vi "Industri Kerupuk Kentang.vi"() -> ()   [LabVIEW 2021]
uses:
  Control 12.ctl
panel:
  out "Proses Packing Selesai":bool
  out "Pencampuran Kentang \ndengan bumbu":bool
  out "Kompor Menyala":bool
  out "Keran 2 Menyala":bool
  out "Proses Pemotongan Kentang":bool
  out "Conveyor 2":dbl(slide)=10.0 scale=0.0..10.0
  out "Closer":dbl(slide) scale=0.0..10.0
  out "Conveyor":dbl(slide)=10.0 scale=0.0..10.0
  out "Pengadukan Bumbu":bool
  out "Pengeringan Bumbu":bool
  out "Tangki Bumbu":dbl(slide) scale=0.0..150.0
  out "Suhu Oven":dbl(slide) scale=0.0..150.0
  out "Silinder single acting":dbl(slide) scale=0.0..2.0
  out "Proximity":bool
  out "Silinder Pemotong 2":dbl(slide) scale=0.0..1.0
  out "Conveyor  2":dbl(slide) scale=0.0..1000.0
  out "Valve":T1
  out "Tachometer":dbl(knob) scale=0.0..250.0
  out "Tangki Minyak":dbl(slide) scale=0.0..1000.0
  out "Tangki Air":dbl(slide) scale=0.0..1000.0
  out "Tangki Penggorengan":dbl(slide) scale=0.0..180.0
  out "Pengukuran berat Kentang":bool
  out "Conveyor  1":dbl(slide) scale=0.0..35.0
  out "Tangki Pencucian":dbl(slide) scale=0.0..180.0
  out "Keran 1 menyala":bool
  out "Suhu Kompor Penggorengan":dbl(slide) scale=0.0..120.0
  out "Kecepatan pengaduk":dbl(knob) scale=0.0..100.0
  out "Berat Kentang":dbl(knob) scale=0.0..100.0
  # "1. Mesin Pengupas Kentang\n(Potato Peeler)"
  # "rpm"
  # "Packing Kerupuk Kentang"
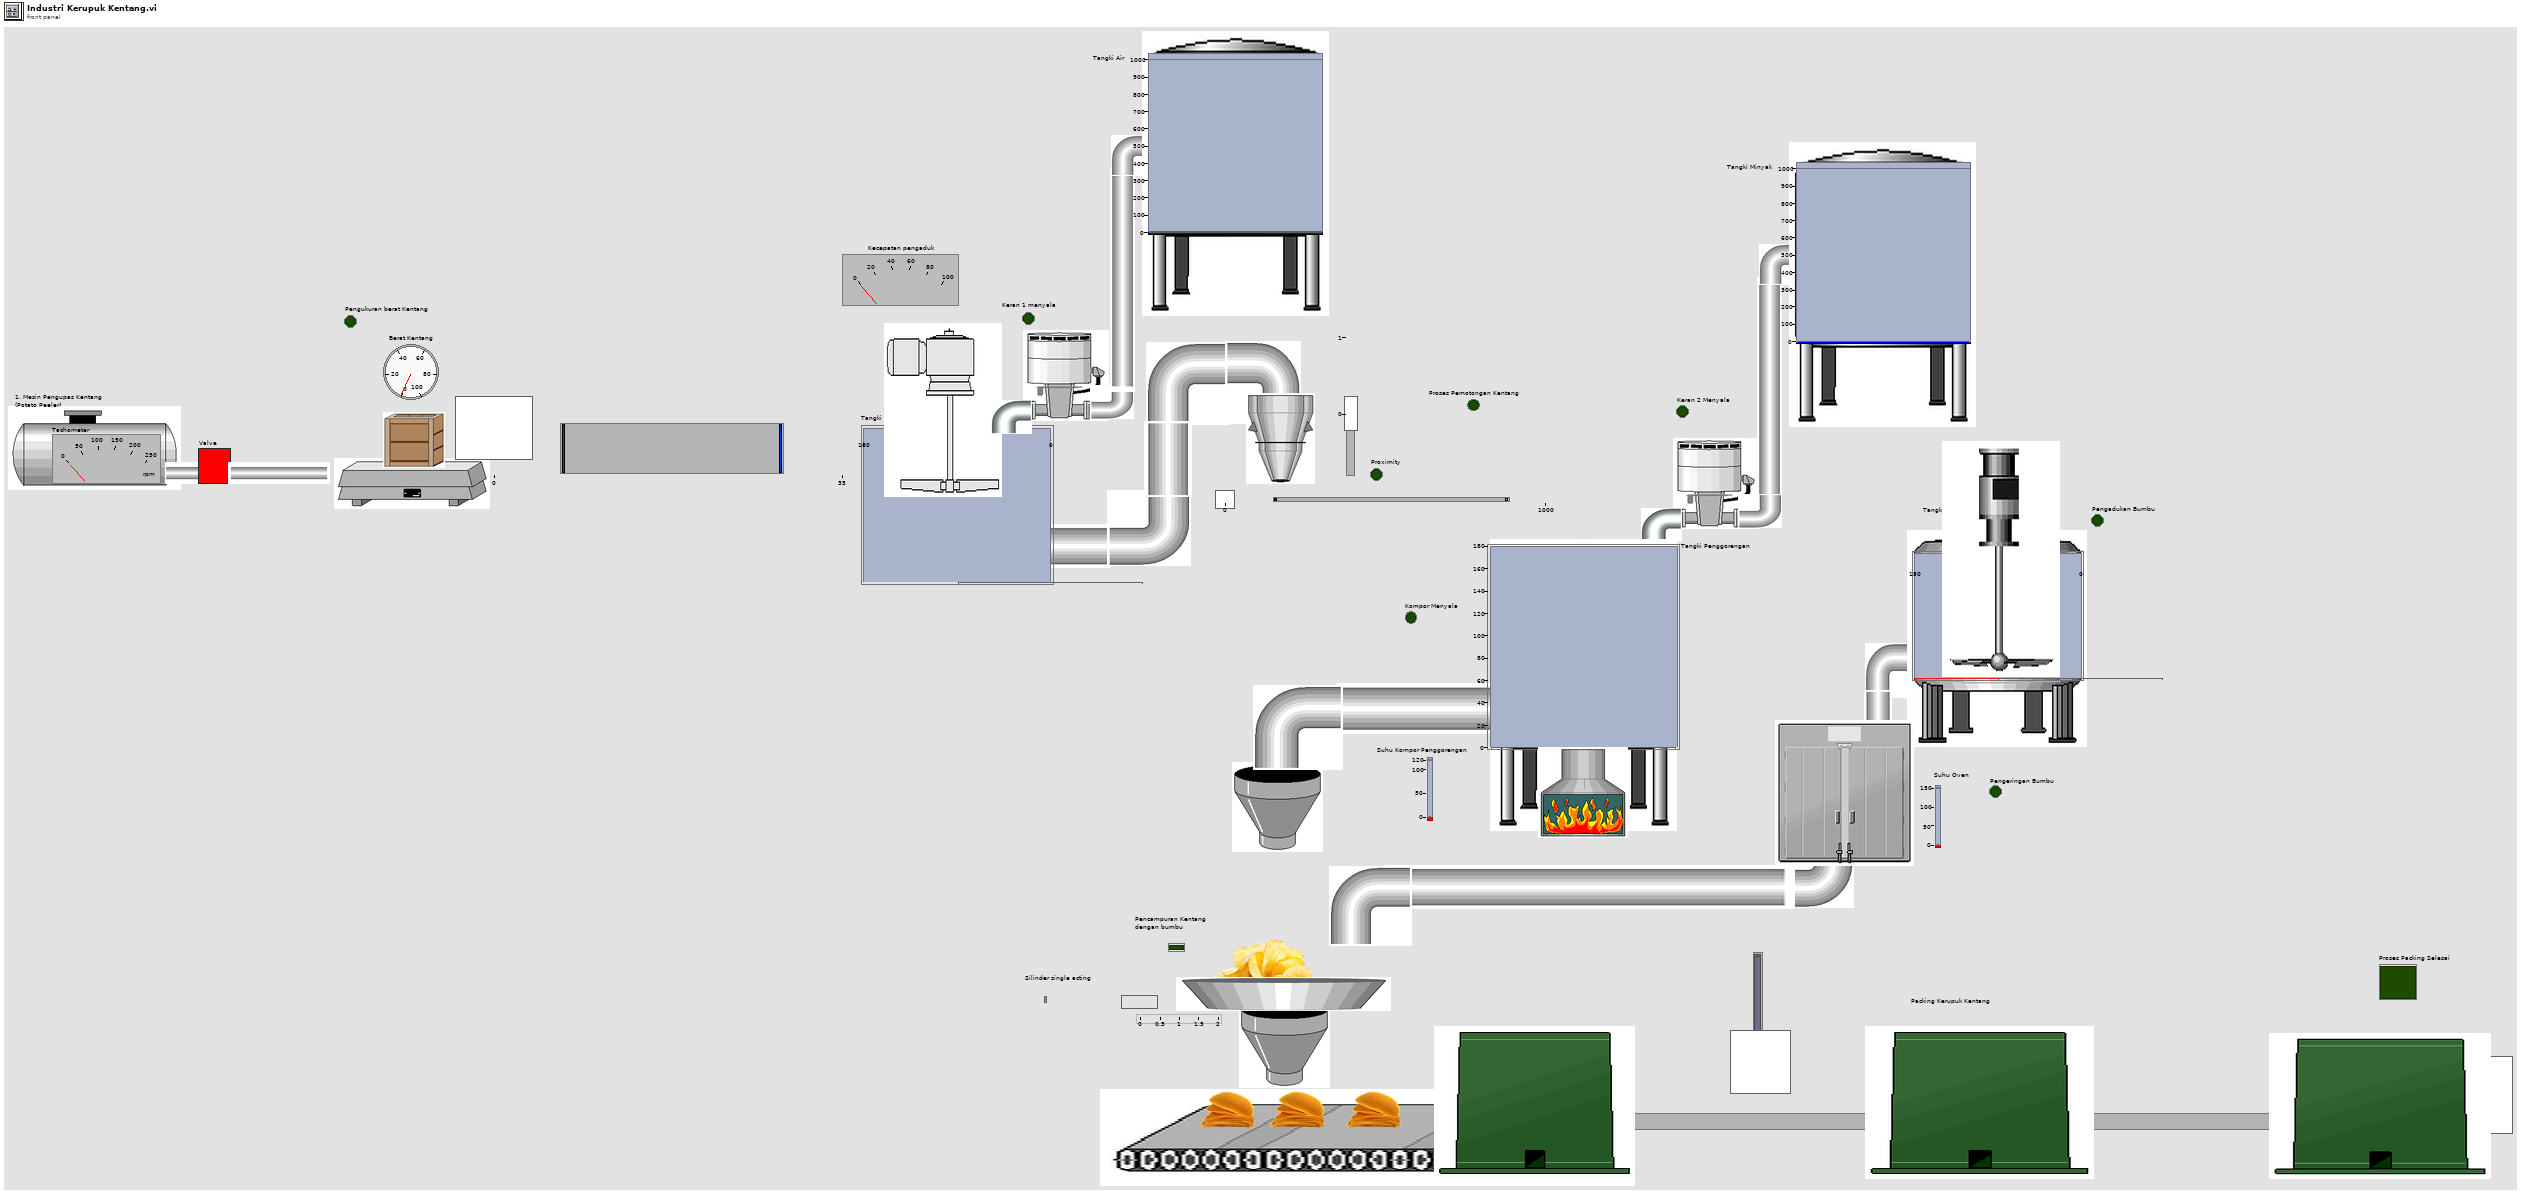
[diagram p1: front panel]
types:
  T1 = typedef "Control 12.ctl" = bool
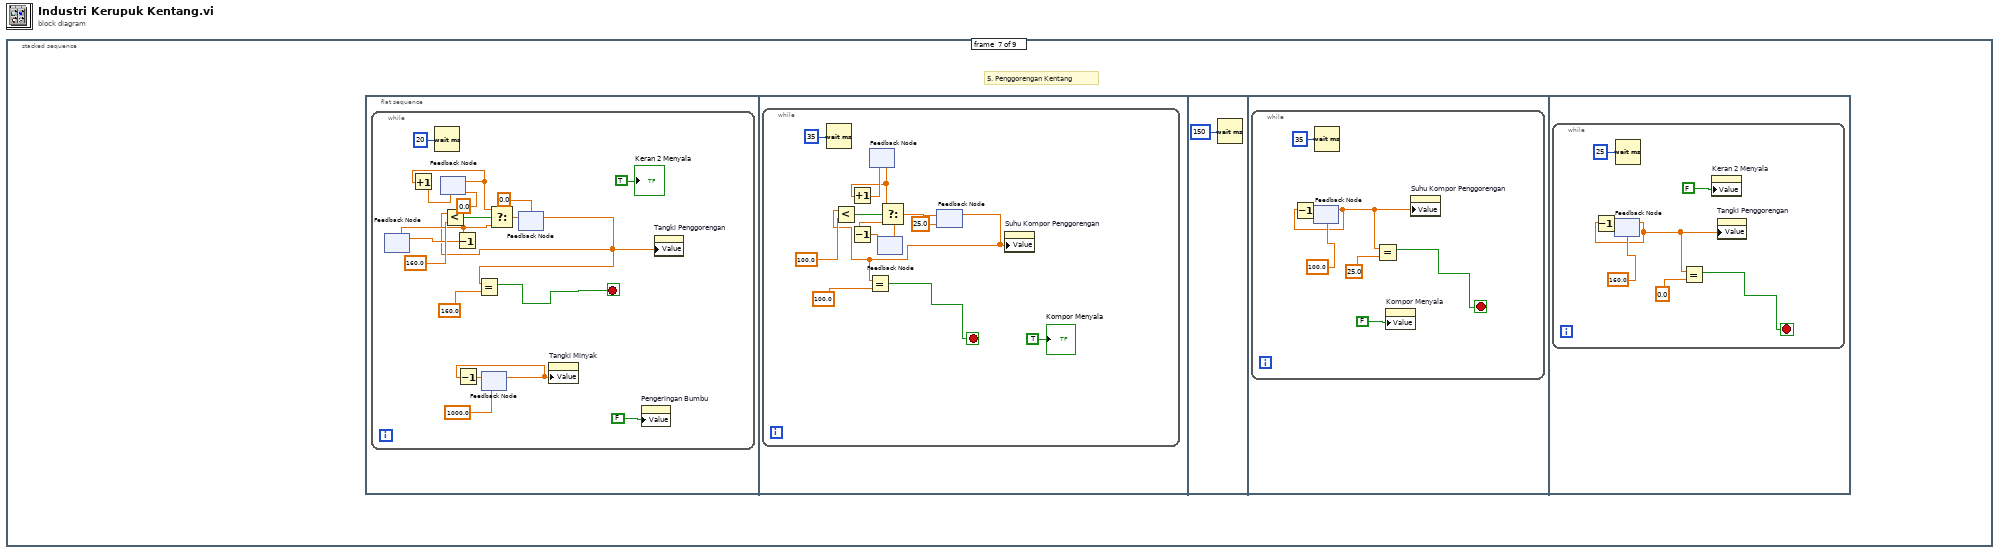
[diagram p0: block diagram]
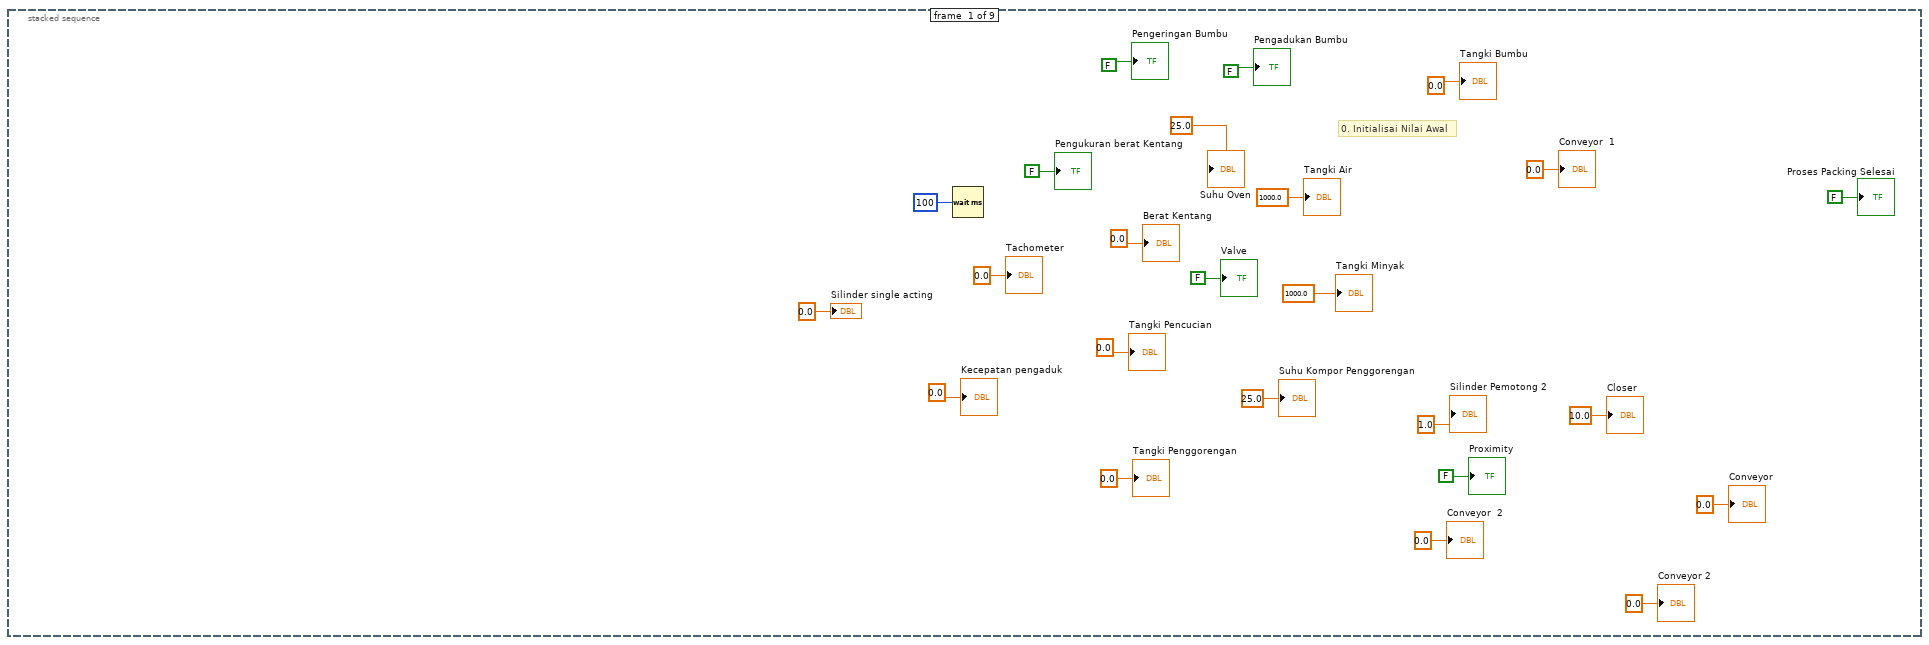
[diagram p2: hidden frame]
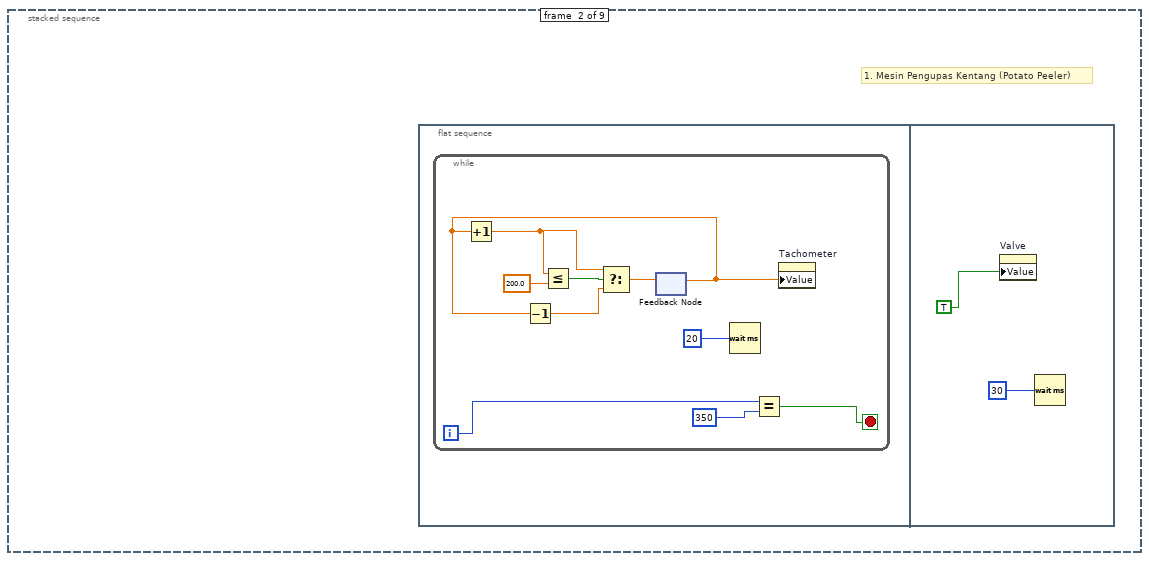
[diagram p3: hidden frame]
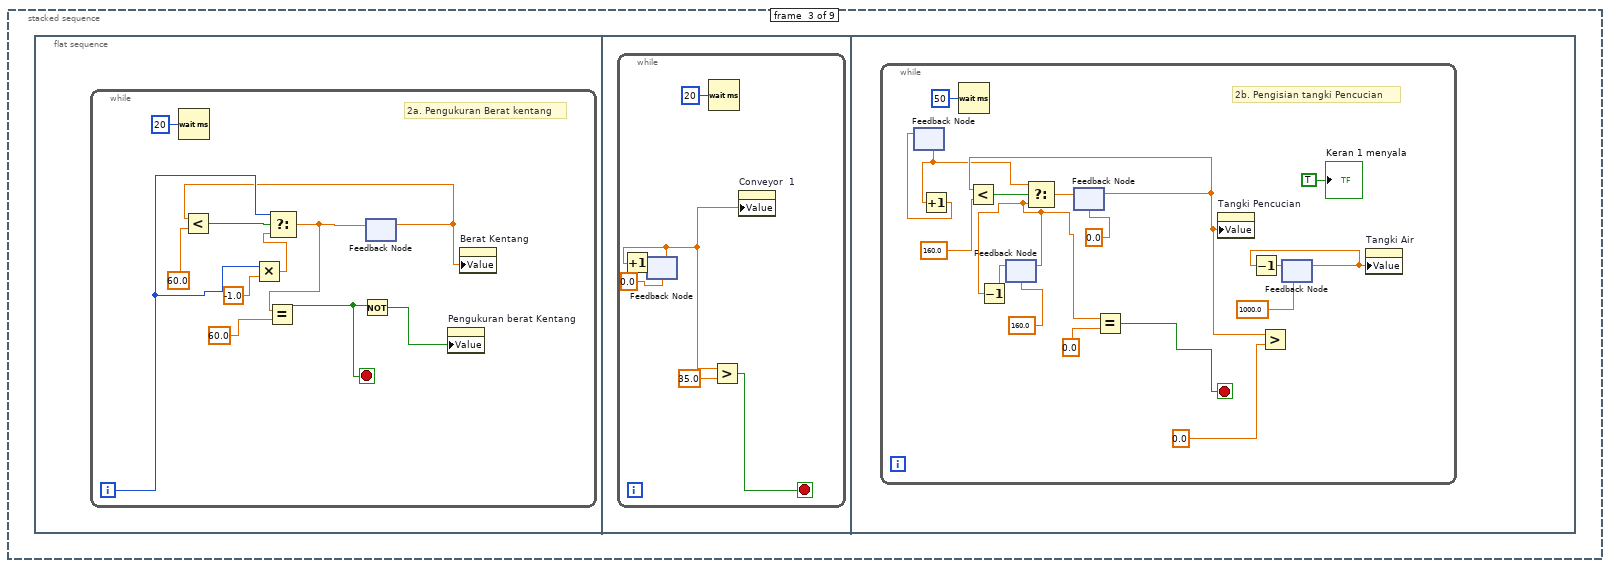
[diagram p4: hidden frame]
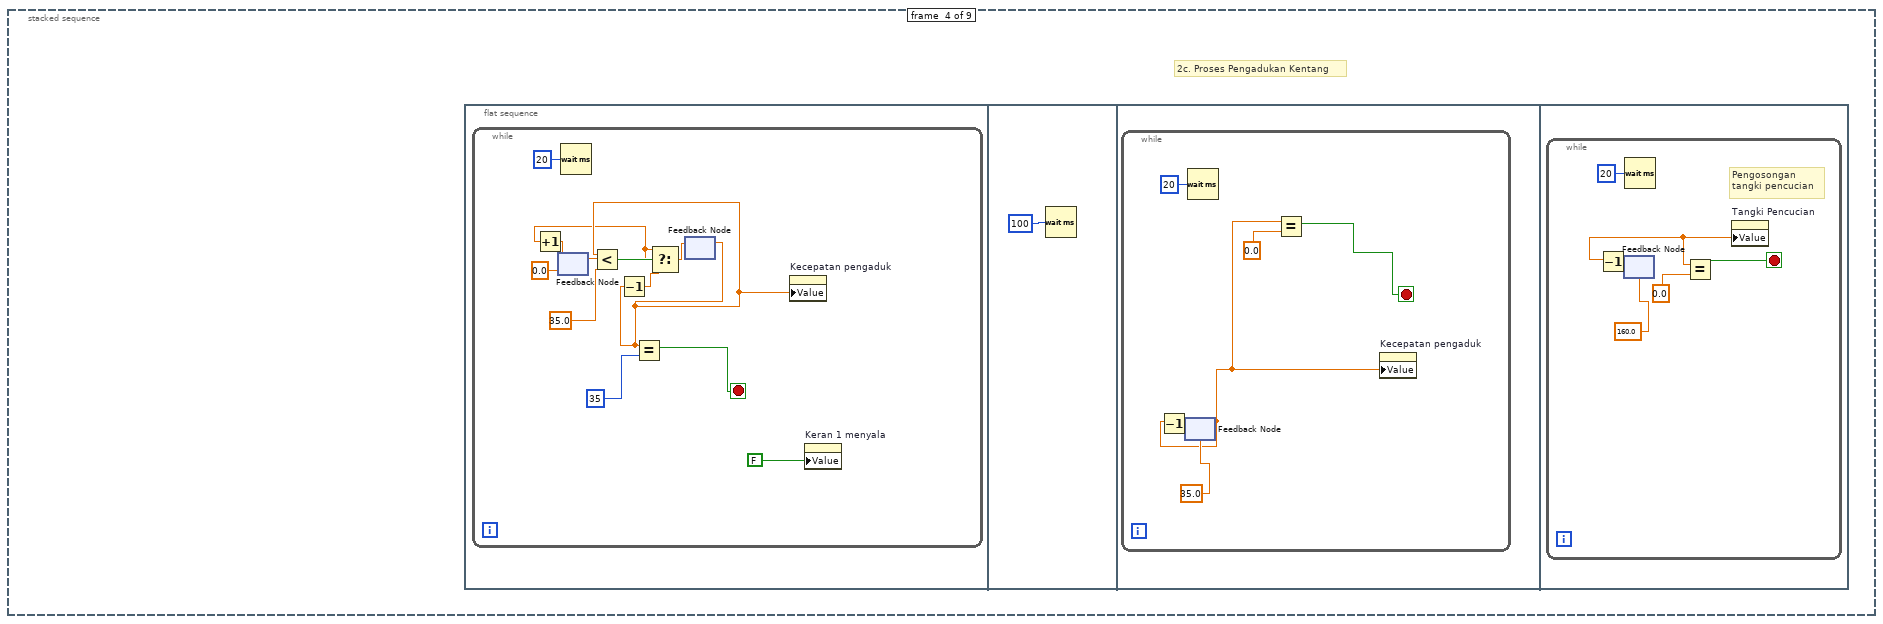
[diagram p5: hidden frame]
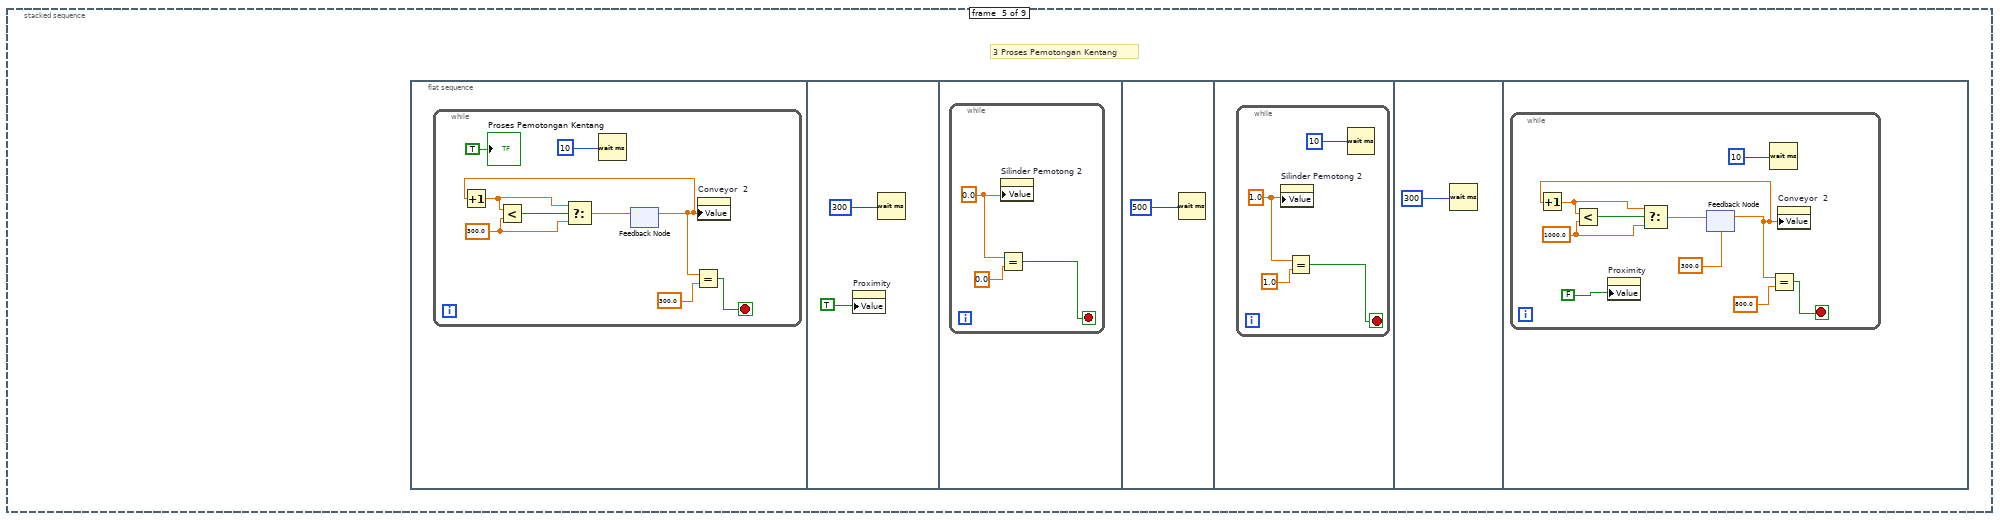
[diagram p6: hidden frame]
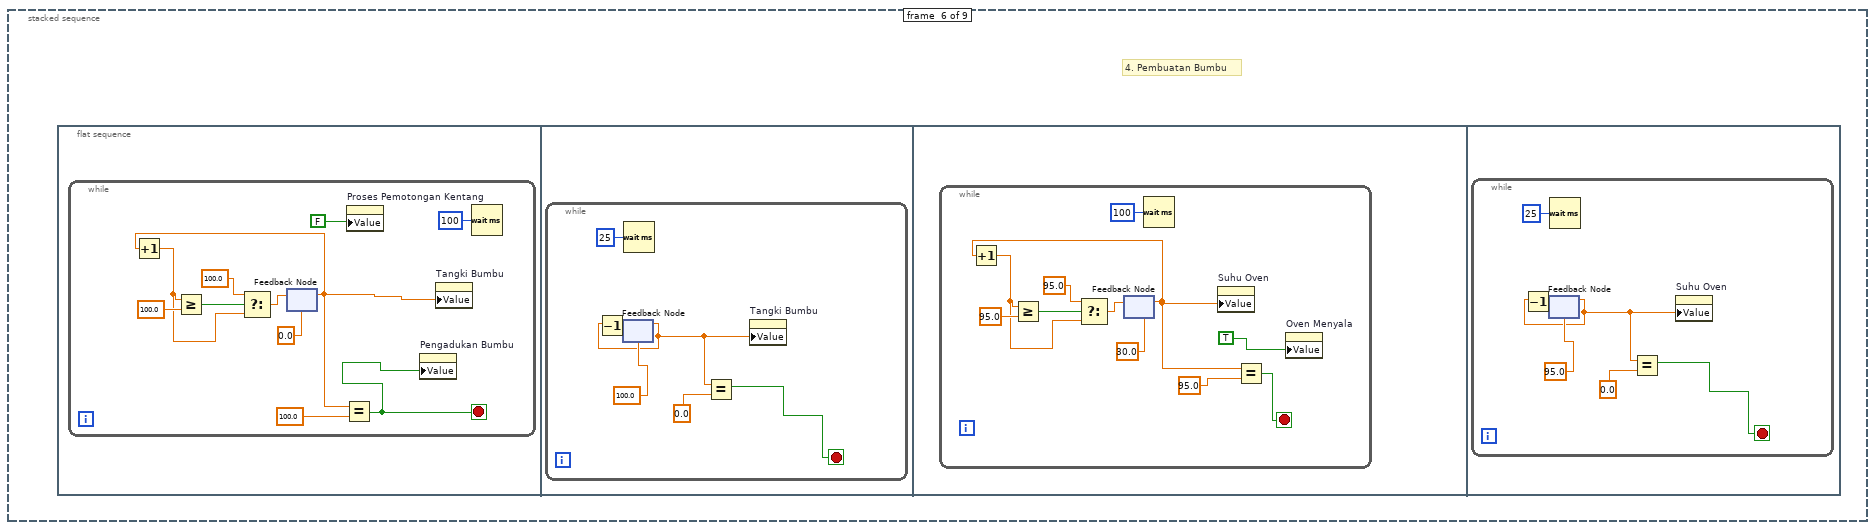
[diagram p7: hidden frame]
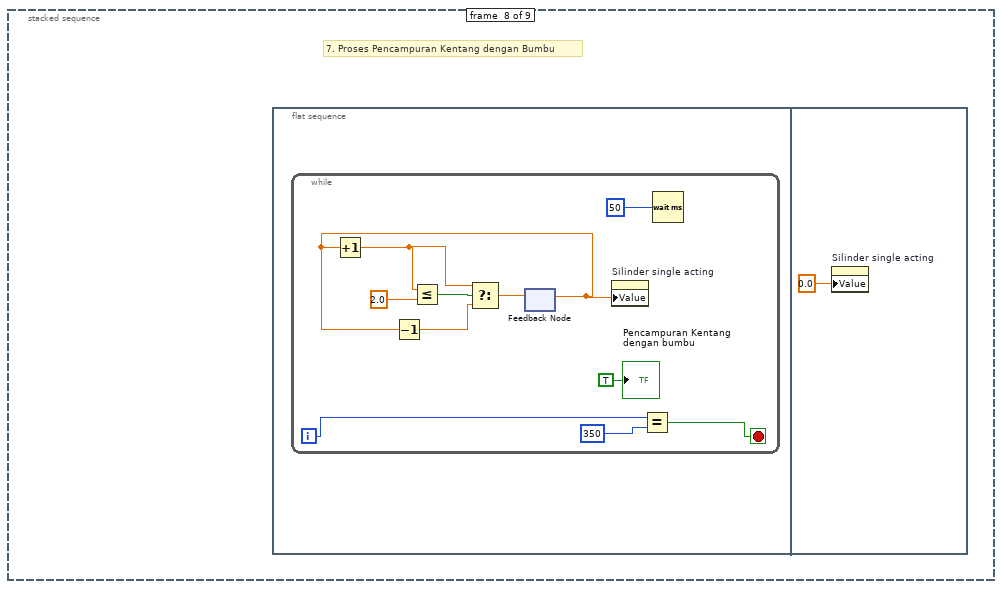
[diagram p8: hidden frame]
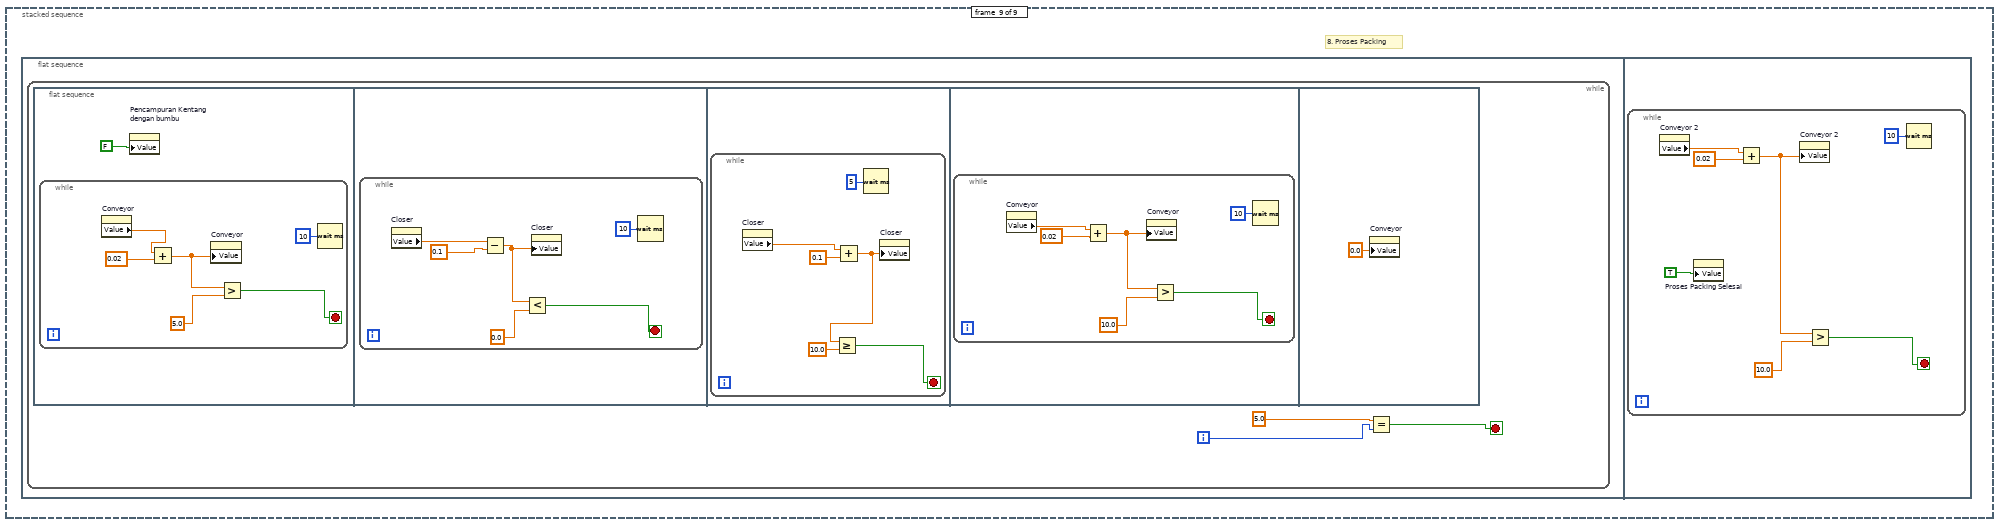
[diagram p9: hidden frame]
diagram:
  n1 = stacked-sequence {
    frame #0 {
      # "0. Initialisai Nilai Awal"
      n2 = Wait (ms)(milliseconds to wait=u32 100) -> ()  [unwired: 1 out]
      "Berat Kentang" <- 0.0 ("Berat Kentang")
      "Tangki Pencucian" <- 0.0 ("Tangki Air 1")
      "Kecepatan pengaduk" <- 0.0 ("Kecepatan pengaduk")
      "Pengukuran berat Kentang" <- FALSE ("Pengukuran berat Kentang")
      "Suhu Kompor Penggorengan" <- 25.0 ("Suhu Kompor Penggorengan")
      "Tangki Penggorengan" <- 0.0 ("Tangki Penggorengan")
      "Tangki Air" <- 1000.0 ("Tangki Air")
      "Tangki Minyak" <- 1000.0 ("Tangki Minyak")
      "Tachometer" <- 0.0 ("Tachometer")
      "Valve" <- T1 FALSE ("Valve")
      "Conveyor  2" <- 0.0 ("Conveyor Kentang 2")
      "Silinder Pemotong 2" <- 1.0 ("Silinder Pemotong 2")
      "Proximity" <- FALSE ("Proximity")
      "Conveyor  1" <- 0.0 ("Conveyor Keripik 4")
      "Silinder single acting" <- 0.0 ("Silinder single acting")
      "Suhu Oven" <- 25.0 ("Temp Tank")
      "Tangki Bumbu" <- 0.0 ("Tangki Bumbu")
      "Pengeringan Bumbu" <- FALSE ("Heating")
      "Pengadukan Bumbu" <- FALSE ("Mixing")
      "Conveyor" <- 0.0 ("Conveyor")
      "Closer" <- 10.0 ("Closer")
      "Conveyor 2" <- 0.0 ("Conveyor 2")
      "Proses Packing Selesai" <- FALSE ("Proses Packing Selesai")
    }
    frame #1 {
      # "1. Mesin Pengupas Kentang (Potato Peeler)"
      n3 = flat-sequence {
        frame #0 {
          n4 = while {
            i -> [w26]
            stop <- w27 stop-if-true
            n5 = feedback #1() -> (w29:dbl)  [unwired: 1 in]
            n6 = Increment(x=w29) -> (x+1=w31:dbl)
            n7 = Decrement(x=w29) -> (x-1=w30:dbl)
            n8 = Less Or Equal?(x=w31, y=200.0) -> (x <= y?=w34:bool)
            n9 = Select(t=w31, s=w34, f=w30) -> (s? t:f=w32:dbl)
            n10 = feedback-in #1(w32) -> ()
            n11 = Wait (ms)(milliseconds to wait=20) -> ()  [unwired: 1 out]
            n12 = Equal?(x=w26, y=350) -> (x = y?=w27:bool)
            n13 = property on="Tachometer" class="Knob (strict)"("Value"=w29) -> ()  [unwired: 2 in, 2 out]
          }
        }
        frame #1 {
          n14 = property on="Valve" class="Bool (strict)"("Value"=TRUE) -> ()  [unwired: 2 in, 2 out]
          n15 = Wait (ms)(milliseconds to wait=30) -> ()  [unwired: 1 out]
        }
      }
    }
    frame #2 {
      n16 = flat-sequence {
        frame #0 {
          n17 = while {
            i -> [w41]
            stop <- w37 stop-if-true
            # "2a. Pengukuran Berat kentang"
            n18 = Wait (ms)(milliseconds to wait=u32 20) -> ()  [unwired: 1 out]
            n19 = Multiply(x=w41, y=-1.0) -> (x*y=w43:dbl)
            n20 = feedback #2() -> (w39:dbl)  [unwired: 1 in]
            n21 = Less?(x=w39, y=60.0) -> (x < y?=w45:bool)
            n22 = Select(t=w41, s=w45, f=w43) -> (s? t:f=w40:dbl)
            n23 = Equal?(x=w40, y=60.0) -> (x = y?=w37:bool)
            n24 = Not(x=w37) -> (.not. x?=w38:bool)
            n25 = feedback-in #2(w40) -> ()
            n26 = property on="Pengukuran berat Kentang" class="Bool (strict)"("Value"=w38) -> ()  [unwired: 2 in, 2 out]
            n27 = property on="Berat Kentang" class="Knob (strict)"("Value"=w39) -> ()  [unwired: 2 in, 2 out]
          }
        }
        frame #1 {
          n28 = while {
            stop <- w49 stop-if-true
            n29 = feedback #3(0.0) -> (w48:dbl)
            n30 = Increment(x=w48) -> (x+1=w51:dbl)
            n31 = feedback-in #3(w51) -> ()
            n32 = Wait (ms)(milliseconds to wait=u32 20) -> ()  [unwired: 1 out]
            n33 = Greater?(x=w48, y=35.0) -> (0:w49:bool)
            n34 = property on="Conveyor  1" class="Slide (strict)"("Value"=w48) -> ()  [unwired: 2 in, 2 out]
          }
        }
        frame #2 {
          n35 = while {
            stop <- w54 stop-if-true
            # "2b. Pengisian tangki Pencucian"
            n36 = feedback #4() -> (w56:dbl)  [unwired: 1 in]
            n37 = Increment(x=w56) -> (x+1=w57:dbl)
            n38 = feedback-in #4(w57) -> ()
            n39 = Wait (ms)(milliseconds to wait=u32 50) -> ()  [unwired: 1 out]
            n40 = feedback #5(160.0) -> (w62:dbl)
            n41 = Decrement(x=w62) -> (x-1=w64:dbl)
            n42 = feedback-in #5(w64) -> ()
            n43 = feedback #6(0.0) -> (w65:dbl)
            n44 = Less?(x=w65, y=160.0) -> (x < y?=w69:bool)
            n45 = Select(t=w56, s=w69, f=w62) -> (s? t:f=w66:dbl)
            n46 = feedback-in #6(w66) -> ()
            n47 = Equal?(x=w62, y=0.0) -> (x = y?=w54:bool)
            n48 = property on="Tangki Pencucian" class="Slide (strict)"("Value"=w65) -> ()  [unwired: 2 in, 2 out]
            n49 = Greater?(x=w65, y=0.0) -> ()  [unwired: 1 out]
            n50 = feedback #7(1000.0) -> (w59:dbl)
            n51 = Decrement(x=w59) -> (x-1=w60:dbl)
            n52 = feedback-in #7(w60) -> ()
            n53 = property on="Tangki Air" class="Slide (strict)"("Value"=w59) -> ()  [unwired: 2 in, 2 out]
            "Keran 1 menyala" <- TRUE ("Keran menyala")
          }
        }
      }
    }
    frame #3 {
      # "2c. Proses Pengadukan Kentang"
      n54 = flat-sequence {
        frame #0 {
          n55 = while {
            stop <- w76 stop-if-true
            n56 = feedback #8(0.0) -> (w73:dbl)
            n57 = Increment(x=w73) -> (x+1=w74:dbl)
            n58 = feedback-in #8(w74) -> ()
            n59 = Wait (ms)(milliseconds to wait=u32 20) -> ()  [unwired: 1 out]
            n60 = feedback #9() -> (w78:dbl)  [unwired: 1 in]
            n61 = Less?(x=w78, y=35.0) -> (x < y?=w80:bool)
            n62 = Decrement(x=w78) -> (x-1=w82:dbl)
            n63 = Equal?(x=w78, y=35) -> (x = y?=w76:bool)
            n64 = Select(t=w73, s=w80, f=w82) -> (s? t:f=w79:dbl)
            n65 = feedback-in #9(w79) -> ()
            n66 = property on="Kecepatan pengaduk" class="Knob (strict)"("Value"=w78) -> ()  [unwired: 2 in, 2 out]
            n67 = property on="Keran 1 menyala" class="Bool (strict)"("Value"=FALSE) -> ()  [unwired: 2 in, 2 out]
          }
        }
        frame #1 {
          n68 = Wait (ms)(milliseconds to wait=u32 100) -> ()  [unwired: 1 out]
        }
        frame #2 {
          n69 = while {
            stop <- w88 stop-if-true
            n70 = feedback #10(35.0) -> (w85:dbl)
            n71 = Decrement(x=w85) -> (x-1=w87:dbl)
            n72 = feedback-in #10(w87) -> ()
            n73 = Wait (ms)(milliseconds to wait=u32 20) -> ()  [unwired: 1 out]
            n74 = Equal?(x=w85, y=0.0) -> (x = y?=w88:bool)
            n75 = property on="Kecepatan pengaduk" class="Knob (strict)"("Value"=w85) -> ()  [unwired: 2 in, 2 out]
          }
        }
        frame #3 {
          n76 = while {
            stop <- w92 stop-if-true
            # "Pengosongan \ntangki pencucian"
            n77 = feedback #11(160.0) -> (w93:dbl)
            n78 = Decrement(x=w93) -> (x-1=w94:dbl)
            n79 = feedback-in #11(w94) -> ()
            n80 = Wait (ms)(milliseconds to wait=u32 20) -> ()  [unwired: 1 out]
            n81 = Equal?(x=w93, y=0.0) -> (x = y?=w92:bool)
            n82 = property on="Tangki Pencucian" class="Slide (strict)"("Value"=w93) -> ()  [unwired: 2 in, 2 out]
          }
        }
      }
    }
    frame #4 {
      # "3 Proses Pemotongan Kentang"
      n83 = flat-sequence {
        frame #0 {
          n84 = while {
            stop <- w101 stop-if-true
            w102 = 300.0
            n85 = Wait (ms)(milliseconds to wait=10) -> ()  [unwired: 1 out]
            n86 = feedback #12() -> (w99:dbl)  [unwired: 1 in]
            n87 = Increment(x=w99) -> (x+1=w103:dbl)
            n88 = Less?(x=w103, y=w102) -> (x < y?=w105:bool)
            n89 = Select(t=w103, s=w105, f=w102) -> (s? t:f=w104:dbl)
            n90 = feedback-in #12(w104) -> ()
            n91 = Equal?(x=w99, y=300.0) -> (x = y?=w101:bool)
            n92 = property on="Conveyor  2" class="Slide (strict)"("Value"=w99) -> ()  [unwired: 2 in, 2 out]
            "Proses Pemotongan Kentang" <- TRUE ("Proses Pemotongan Kentang")
          }
        }
        frame #1 {
          n93 = property on="Proximity" class="Bool (strict)"("Value"=TRUE) -> ()  [unwired: 2 in, 2 out]
          n94 = Wait (ms)(milliseconds to wait=300) -> ()  [unwired: 1 out]
        }
        frame #2 {
          n95 = while {
            stop <- w108 stop-if-true
            w109 = 0.0
            n96 = Equal?(x=w109, y=0.0) -> (x = y?=w108:bool)
            n97 = property on="Silinder Pemotong 2" class="Slide (strict)"("Value"=w109) -> ()  [unwired: 2 in, 2 out]
          }
        }
        frame #3 {
          n98 = Wait (ms)(milliseconds to wait=500) -> ()  [unwired: 1 out]
        }
        frame #4 {
          n99 = while {
            stop <- w113 stop-if-true
            w114 = 1.0
            n100 = property on="Silinder Pemotong 2" class="Slide (strict)"("Value"=w114) -> ()  [unwired: 2 in, 2 out]
            n101 = Equal?(x=w114, y=1.0) -> (x = y?=w113:bool)
            n102 = Wait (ms)(milliseconds to wait=10) -> ()  [unwired: 1 out]
          }
        }
        frame #5 {
          n103 = Wait (ms)(milliseconds to wait=300) -> ()  [unwired: 1 out]
        }
        frame #6 {
          n104 = while {
            stop <- w122 stop-if-true
            w123 = 1000.0
            n105 = property on="Proximity" class="Bool (strict)"("Value"=FALSE) -> ()  [unwired: 2 in, 2 out]
            n106 = feedback #13(300.0) -> (w120:dbl)
            n107 = Increment(x=w120) -> (x+1=w124:dbl)
            n108 = Less?(x=w124, y=w123) -> (x < y?=w126:bool)
            n109 = Select(t=w124, s=w126, f=w123) -> (s? t:f=w125:dbl)
            n110 = feedback-in #13(w125) -> ()
            n111 = Wait (ms)(milliseconds to wait=10) -> ()  [unwired: 1 out]
            n112 = Equal?(x=w120, y=800.0) -> (x = y?=w122:bool)
            n113 = property on="Conveyor  2" class="Slide (strict)"("Value"=w120) -> ()  [unwired: 2 in, 2 out]
          }
        }
      }
    }
    frame #5 {
      # "4. Pembuatan Bumbu"
      n114 = flat-sequence {
        frame #0 {
          n115 = while {
            stop <- w128 stop-if-true
            n116 = feedback #14(0.0 ("t")) -> (w129:dbl)
            n117 = Increment(x=w129) -> (x+1=w131:dbl)
            n118 = Greater Or Equal?(x=w131, y=100.0) -> (x >= y?=w135:bool)
            n119 = Select(t=100.0, s=w135, f=w131) -> (s? t:f=w132:dbl)
            n120 = feedback-in #14(w132) -> ()
            n121 = Equal?(x=w129, y=100.0) -> (x = y?=w128:bool)
            n122 = property on="Proses Pemotongan Kentang" class="Bool (strict)"("Value"=FALSE) -> ()  [unwired: 2 in, 2 out]
            n123 = property on="Pengadukan Bumbu" class="Bool (strict)"("Value"=w128) -> ()  [unwired: 2 in, 2 out]
            n124 = property on="Tangki Bumbu" class="Slide (strict)"("Value"=w129) -> ()  [unwired: 2 in, 2 out]
            n125 = Wait (ms)(milliseconds to wait=u32 100) -> ()  [unwired: 1 out]
          }
        }
        frame #1 {
          n126 = while {
            stop <- w140 stop-if-true
            n127 = feedback #15(100.0) -> (w138:dbl)
            n128 = Decrement(x=w138) -> (x-1=w141:dbl)
            n129 = feedback-in #15(w141) -> ()
            n130 = Wait (ms)(milliseconds to wait=u32 25) -> ()  [unwired: 1 out]
            n131 = Equal?(x=w138, y=0.0) -> (x = y?=w140:bool)
            n132 = property on="Tangki Bumbu" class="Slide (strict)"("Value"=w138) -> ()  [unwired: 2 in, 2 out]
          }
        }
        frame #2 {
          n133 = while {
            stop <- w147 stop-if-true
            n134 = feedback #16(30.0 ("t")) -> (w145:dbl)
            n135 = Increment(x=w145) -> (x+1=w148:dbl)
            n136 = Greater Or Equal?(x=w148, y=95.0) -> (x >= y?=w151:bool)
            n137 = Select(t=95.0, s=w151, f=w148) -> (s? t:f=w149:dbl)
            n138 = feedback-in #16(w149) -> ()
            n139 = Wait (ms)(milliseconds to wait=u32 100) -> ()  [unwired: 1 out]
            n140 = property on="Suhu Oven" class="Slide (strict)"("Value"=w145) -> ()  [unwired: 2 in, 2 out]
            n141 = Equal?(x=w145, y=95.0) -> (x = y?=w147:bool)
            n142 = property on="Oven Menyala" class="Bool (strict)"("Value"=TRUE ("Heating")) -> ()  [unwired: 2 in, 2 out]
          }
        }
        frame #3 {
          n143 = while {
            stop <- w157 stop-if-true
            n144 = feedback #17(95.0) -> (w155:dbl)
            n145 = Decrement(x=w155) -> (x-1=w158:dbl)
            n146 = feedback-in #17(w158) -> ()
            n147 = Wait (ms)(milliseconds to wait=u32 25) -> ()  [unwired: 1 out]
            n148 = Equal?(x=w155, y=0.0) -> (x = y?=w157:bool)
            n149 = property on="Suhu Oven" class="Slide (strict)"("Value"=w155) -> ()  [unwired: 2 in, 2 out]
          }
        }
      }
    }
    frame #6 {
      # "5. Penggorengan Kentang"
      n150 = flat-sequence {
        frame #0 {
          n151 = while {
            stop <- w171 stop-if-true
            n152 = feedback #18() -> (w165:dbl)  [unwired: 1 in]
            n153 = Wait (ms)(milliseconds to wait=u32 20) -> ()  [unwired: 1 out]
            n154 = feedback #19(0.0) -> (w169:dbl)
            n155 = Increment(x=w169) -> (x+1=w170:dbl)
            n156 = feedback-in #19(w170) -> ()
            n157 = Decrement(x=w165) -> (x-1=w166:dbl)
            n158 = feedback-in #18(w166) -> ()
            n159 = feedback #20(1000.0) -> (w173:dbl)
            n160 = Decrement(x=w173) -> (x-1=w174:dbl)
            n161 = feedback-in #20(w174) -> ()
            n162 = feedback #21(0.0) -> (w164:dbl)
            n163 = Less?(x=w164, y=160.0) -> (x < y?=w176:bool)
            n164 = Equal?(x=w164, y=160.0) -> (x = y?=w171:bool)
            n165 = Select(t=w169, s=w176, f=w165) -> (s? t:f=w167:dbl)
            n166 = feedback-in #21(w167) -> ()
            n167 = property on="Tangki Minyak" class="Slide (strict)"("Value"=w173) -> ()  [unwired: 2 in, 2 out]
            n168 = property on="Pengeringan Bumbu" class="Bool (strict)"("Value"=FALSE) -> ()  [unwired: 2 in, 2 out]
            n169 = property on="Tangki Penggorengan" class="Slide (strict)"("Value"=w164) -> ()  [unwired: 2 in, 2 out]
            "Keran 2 Menyala" <- TRUE ("Keran 2")
          }
        }
        frame #1 {
          n170 = while {
            stop <- w180 stop-if-true
            n171 = Wait (ms)(milliseconds to wait=u32 35) -> ()  [unwired: 1 out]
            n172 = feedback #22() -> (w186:dbl)  [unwired: 1 in]
            n173 = Increment(x=w186) -> (x+1=w187:dbl)
            n174 = feedback-in #22(w187) -> ()
            n175 = feedback #23() -> (w184:dbl)  [unwired: 1 in]
            n176 = Decrement(x=w184) -> (x-1=w185:dbl)
            n177 = feedback-in #23(w185) -> ()
            n178 = feedback #24(25.0) -> (w182:dbl)
            n179 = Less?(x=w182, y=100.0) -> (x < y?=w189:bool)
            n180 = Equal?(x=w182, y=100.0) -> (x = y?=w180:bool)
            n181 = Select(t=w186, s=w189, f=w184) -> (s? t:f=w183:dbl)
            n182 = feedback-in #24(w183) -> ()
            n183 = property on="Suhu Kompor Penggorengan" class="Slide (strict)"("Value"=w182) -> ()  [unwired: 2 in, 2 out]
            "Kompor Menyala" <- TRUE ("Kompor Menyala")
          }
        }
        frame #2 {
          n184 = Wait (ms)(milliseconds to wait=u32 150) -> ()  [unwired: 1 out]
        }
        frame #3 {
          n185 = while {
            stop <- w196 stop-if-true
            n186 = feedback #25(100.0) -> (w194:dbl)
            n187 = Decrement(x=w194) -> (x-1=w197:dbl)
            n188 = feedback-in #25(w197) -> ()
            n189 = Wait (ms)(milliseconds to wait=u32 35) -> ()  [unwired: 1 out]
            n190 = Equal?(x=w194, y=25.0) -> (x = y?=w196:bool)
            n191 = property on="Kompor Menyala" class="Bool (strict)"("Value"=FALSE) -> ()  [unwired: 2 in, 2 out]
            n192 = property on="Suhu Kompor Penggorengan" class="Slide (strict)"("Value"=w194) -> ()  [unwired: 2 in, 2 out]
          }
        }
        frame #4 {
          n193 = while {
            stop <- w203 stop-if-true
            n194 = feedback #26(160.0) -> (w201:dbl)
            n195 = Decrement(x=w201) -> (x-1=w204:dbl)
            n196 = feedback-in #26(w204) -> ()
            n197 = Wait (ms)(milliseconds to wait=u32 25) -> ()  [unwired: 1 out]
            n198 = Equal?(x=w201, y=0.0) -> (x = y?=w203:bool)
            n199 = property on="Keran 2 Menyala" class="Bool (strict)"("Value"=FALSE) -> ()  [unwired: 2 in, 2 out]
            n200 = property on="Tangki Penggorengan" class="Slide (strict)"("Value"=w201) -> ()  [unwired: 2 in, 2 out]
          }
        }
      }
    }
    frame #7 {
      # "7. Proses Pencampuran Kentang dengan Bumbu"
      n201 = flat-sequence {
        frame #0 {
          n202 = while {
            i -> [w209]
            stop <- w210 stop-if-true
            n203 = feedback #27() -> (w212:dbl)  [unwired: 1 in]
            n204 = Increment(x=w212) -> (x+1=w214:dbl)
            n205 = Decrement(x=w212) -> (x-1=w213:dbl)
            n206 = Less Or Equal?(x=w214, y=2.0) -> (x <= y?=w217:bool)
            n207 = Select(t=w214, s=w217, f=w213) -> (s? t:f=w215:dbl)
            n208 = feedback-in #27(w215) -> ()
            n209 = property on="Silinder single acting" class="Slide (strict)"("Value"=w212) -> ()  [unwired: 2 in, 2 out]
            n210 = Equal?(x=w209, y=350) -> (x = y?=w210:bool)
            n211 = Wait (ms)(milliseconds to wait=50) -> ()  [unwired: 1 out]
            "Pencampuran Kentang \ndengan bumbu" <- TRUE ("Pencampuran Kentang \ndengan bumbu")
          }
        }
        frame #1 {
          n212 = property on="Silinder single acting" class="Slide (strict)"("Value"=0.0) -> ()  [unwired: 2 in, 2 out]
        }
      }
    }
    frame #8 {
      # "8. Proses Packing"
      n213 = flat-sequence {
        frame #0 {
          n214 = while {
            i -> [w221]
            stop <- w219 stop-if-true
            n215 = flat-sequence {
              frame #0 {
                n216 = while {
                  stop <- w223 stop-if-true
                  n217 = property on="Conveyor" class="Slide (strict)"() -> ("Value"=w227:dbl)  [unwired: 2 in, 2 out]
                  n218 = Add(x=w227, y=0.02) -> (x+y=w225:dbl)
                  n219 = property on="Conveyor" class="Slide (strict)"("Value"=w225) -> ()  [unwired: 2 in, 2 out]
                  n220 = Greater?(x=w225, y=5.0) -> (0:w223:bool)
                  n221 = Wait (ms)(milliseconds to wait=u32 10) -> ()  [unwired: 1 out]
                }
                n222 = property on="Pencampuran Kentang \ndengan bumbu" class="Bool (strict)"("Value"=FALSE) -> ()  [unwired: 2 in, 2 out]
              }
              frame #1 {
                n223 = while {
                  stop <- w233 stop-if-true
                  n224 = property on="Closer" class="Slide (strict)"() -> ("Value"=w231:dbl)  [unwired: 2 in, 2 out]
                  n225 = Subtract(x=w231, y=0.1) -> (x-y=w229:dbl)
                  n226 = Less?(x=w229, y=0.0) -> (x < y?=w233:bool)
                  n227 = property on="Closer" class="Slide (strict)"("Value"=w229) -> ()  [unwired: 2 in, 2 out]
                  n228 = Wait (ms)(milliseconds to wait=u32 10) -> ()  [unwired: 1 out]
                }
              }
              frame #2 {
                n229 = while {
                  stop <- w238 stop-if-true
                  n230 = property on="Closer" class="Slide (strict)"() -> ("Value"=w236:dbl)  [unwired: 2 in, 2 out]
                  n231 = Add(x=w236, y=0.1) -> (x+y=w237:dbl)
                  n232 = Greater Or Equal?(x=w237, y=10.0) -> (x >= y?=w238:bool)
                  n233 = Wait (ms)(milliseconds to wait=u32 5) -> ()  [unwired: 1 out]
                  n234 = property on="Closer" class="Slide (strict)"("Value"=w237) -> ()  [unwired: 2 in, 2 out]
                }
              }
              frame #3 {
                n235 = while {
                  stop <- w241 stop-if-true
                  n236 = property on="Conveyor" class="Slide (strict)"() -> ("Value"=w245:dbl)  [unwired: 2 in, 2 out]
                  n237 = Add(x=w245, y=0.02) -> (x+y=w243:dbl)
                  n238 = property on="Conveyor" class="Slide (strict)"("Value"=w243) -> ()  [unwired: 2 in, 2 out]
                  n239 = Greater?(x=w243, y=10.0) -> (0:w241:bool)
                  n240 = Wait (ms)(milliseconds to wait=u32 10) -> ()  [unwired: 1 out]
                }
              }
              frame #4 {
                n241 = property on="Conveyor" class="Slide (strict)"("Value"=0.0 ("Conveyor")) -> ()  [unwired: 2 in, 2 out]
              }
            }
            n242 = Equal?(x=5.0 ("y"), y=w221) -> (x = y?=w219:bool)
          }
        }
        frame #1 {
          n243 = while {
            stop <- w249 stop-if-true
            n244 = property on="Conveyor 2" class="Slide (strict)"() -> ("Value"=w253:dbl)  [unwired: 2 in, 2 out]
            n245 = property on="Proses Packing Selesai" class="Bool (strict)"("Value"=TRUE) -> ()  [unwired: 2 in, 2 out]
            n246 = Add(x=w253, y=0.02) -> (x+y=w251:dbl)
            n247 = property on="Conveyor 2" class="Slide (strict)"("Value"=w251) -> ()  [unwired: 2 in, 2 out]
            n248 = Greater?(x=w251, y=10.0) -> (0:w249:bool)
            n249 = Wait (ms)(milliseconds to wait=u32 10) -> ()  [unwired: 1 out]
          }
        }
      }
    }
  }
